vi "Store XY.vi"(8 "error in (no error)":errorcluster, 11 "Cursor Digitizer in":refnum<class "Cursor Digitizer.lvclass">) -> (0 "error out":errorcluster, 3 "Cursor Digitizer out":refnum<class "Cursor Digitizer.lvclass">)   [LabVIEW 2019, in "Cursor Digitizer.lvclass"]
uses:
  Cursor Digitizer.lvclass
  Cursor Digitizer.lvclass/Cursor Digitizer.ctl
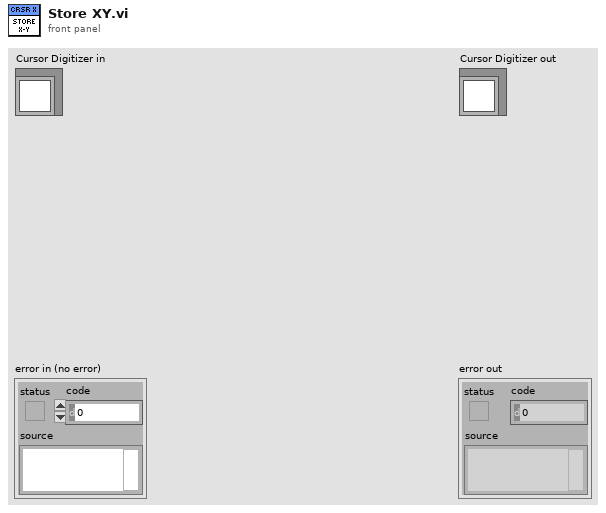
[diagram p1: front panel]
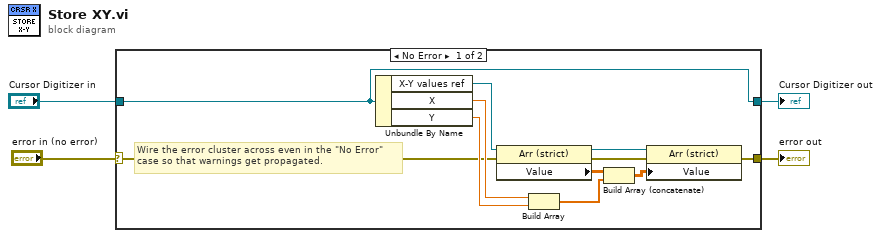
[diagram p0: block diagram]
diagram:
  n1 = case shown="No Error" "error in (no error)" {
    selector: "error in (no error)" -> [w6 w17]
    tunnel: [w5 w17] -> w3
    tunnel: [w15 w16] -> w1
    tunnel: "Cursor Digitizer in" -> [w15 w16]
    frame No Error {
      # "Wire the error cluster across even in the \"No Error\"\ncase so that warnings get propagated."
      n2 = Unbundle By Name(w15) -> ("X-Y values ref"=w14:refnum<vi>, "X"=w12:dbl, "Y"=w11:dbl)
      n3 = property class="Arr (strict)"(reference=w14, error in=w6) -> (reference out=w9:refnum<vi>, error out=w7:errorcluster, "Value"=w13:dbl[][])
      n4 = Build Array(w12, w11) -> (w10:dbl[])
      n5 = Build Array (concatenate)(w13, w10) -> (w8:dbl[][])
      n6 = property class="Arr (strict)"(reference=w9, error in=w7, "Value"=w8) -> (error out=w5:errorcluster)  [unwired: 1 out]
    }
    frame Error {
    }
  }
  "error out" <- w3
  "Cursor Digitizer out" <- w1
